vi "替换数组子集函数1.vi"() -> ()   [LabVIEW 2012]
panel:
  out "输出数组":i32[](array[numeric])
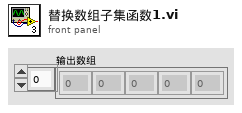
[diagram p1: front panel]
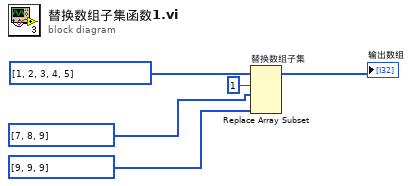
[diagram p0: block diagram]
diagram:
  n1 = Replace Array Subset "替换数组子集"(array=i32[] [1, 2, 3, 4, 5], new element #1=i32[] [7, 8, 9], index #1=1 ("索引"), new element #2=i32[] [9, 9, 9]) -> (→"输出数组":i32[])  [unwired: 1 in]
